vi "rwfm_CustomErrors.vi"() -> (2 "Error Array":errorcluster[](array[cluster])=[{"status"=TRUE, "code"=-5000, "source"="rwfm_Read(poly).vi<ERR>Read Timeout:  This error happens if the Read VI does not receive all the requested samples before the user specified timeout period.  Make sure the FPGA VI was started or increase the timeout. "}, {"status"=TRUE, "code"=-5001, "source"="rwfm_Read(poly).vi<ERR>cRIO Module Underflow:  This error happens if post-processing code on the FPGA VI cannot execute in one acquisition period.  You must lower your sample rate or reduce the amount of post-processing performed on the FPGA."}, {"status"=TRUE, "code"=-5002, "source"="rwfm_Read(poly).vi<ERR>FPGA DMA Overflow:  This error happens if the host application cannot keep up with the DMA transfer and the RT data buffer completely fills up.  Lower your sample rate, increase your samples to read, reduce your CPU usage, or switch to a finite acquisition. "}, {"status"=TRUE, "code"=-5003, "source"="rwfm_Read(poly).vi<ERR>Incorrect Channel Count:  The number of channels specified by rwfm_CreateChan.vi must equal the number of channels in the FPGA VI."}])   [LabVIEW 2017, in "cRIOWfmLib.lvlib"]
uses:
  <vilib>/addons/InsightCM/Devices/Shared/Cms/cRIOWfmAcq/cRIOWfmLib.lvlib
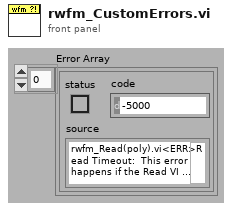
[diagram p1: front panel]
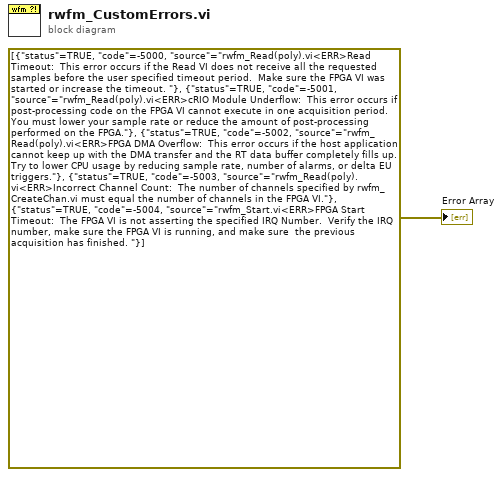
[diagram p0: block diagram]
diagram:
  "Error Array" <- errorcluster[] [{"status"=TRUE, "code"=-5000, "source"="rwfm_Read(poly).vi<ERR>Read Timeout:  This error occurs if the Read VI does not receive all the requested samples before the user specified timeout period.  Make sure the FPGA VI was started or increase the timeout. "}, {"status"=TRUE, "code"=-5001, "source"="rwfm_Read(poly).vi<ERR>cRIO Module Underflow:  This error occurs if post-processing code on the FPGA VI cannot execute in one acquisition period.  You must lower your sample rate or reduce the amount of post-processing performed on the FPGA."}, {"status"=TRUE, "code"=-5002, "source"="rwfm_Read(poly).vi<ERR>FPGA DMA Overflow:  This error occurs if the host application cannot keep up with the DMA transfer and the RT data buffer completely fills up.  Try to lower CPU usage by reducing sample rate, number of alarms, or delta EU triggers."}, {"status"=TRUE, "code"=-5003, "source"="rwfm_Read(poly).vi<ERR>Incorrect Channel Count:  The number of channels specified by rwfm_CreateChan.vi must equal the number of channels in the FPGA VI."}, {"status"=TRUE, "code"=-5004, "source"="rwfm_Start.vi<ERR>FPGA Start Timeout:  The FPGA VI is not asserting the specified IRQ Number.  Verify the IRQ number, make sure the FPGA VI is running, and make sure  the previous acquisition has finished. "}]
